vi "Do Start.vi"(6 "Diagnostics Queue":refnum<queue>, 7 "Host Resources":T1, 8 "error in":errorcluster, 10 "Generated Data":string, 11 "Hardware Configuration in":T5) -> (0 "error out":errorcluster, 2 "Acquired Data":T4, 3 "Hardware Configuration out":T5)   [LabVIEW 2021, in "Load Frame.lvlib"]
doc: "Configure DAQmx tasks to take measurements from the Load Frame sensors using the settings from 'Hardware Configuration in'."
uses:
  Load Frame.lvlib
  Acquisition/Hardware Configuration.ctl
  Acquisition/Channel Settings.ctl
  Acquisition/IO Device.ctl
  Acquisition/Sensor Type.ctl
  Interval Timer/Repeat Interval.ctl
  Interval Timer/Interval Length.ctl
  Interval Timer/Interval Token.ctl
  Acquisition/IO Context.ctl
  Acquisition/IO API.ctl
  Acquisition/Acquired Data.ctl
  Acquisition/Host Resources.ctl
  Acquisition/Host Software Package.ctl
  Acquisition/Host IO Resource.ctl
  support/Message Queue/Message Cluster.ctl
  74e49535-f2c9-4e2d-86ae-5e165b5420e6.vi
  c62da056-855e-47fb-b67a-8cab6a77d309.vi
  support/Message Queue/Enqueue Message (Single).vi
  support/Message Queue/Message Queue.lvlib
  Acquisition/Acquisition.lvlib
  Interval Timer/Interval Timer.lvlib
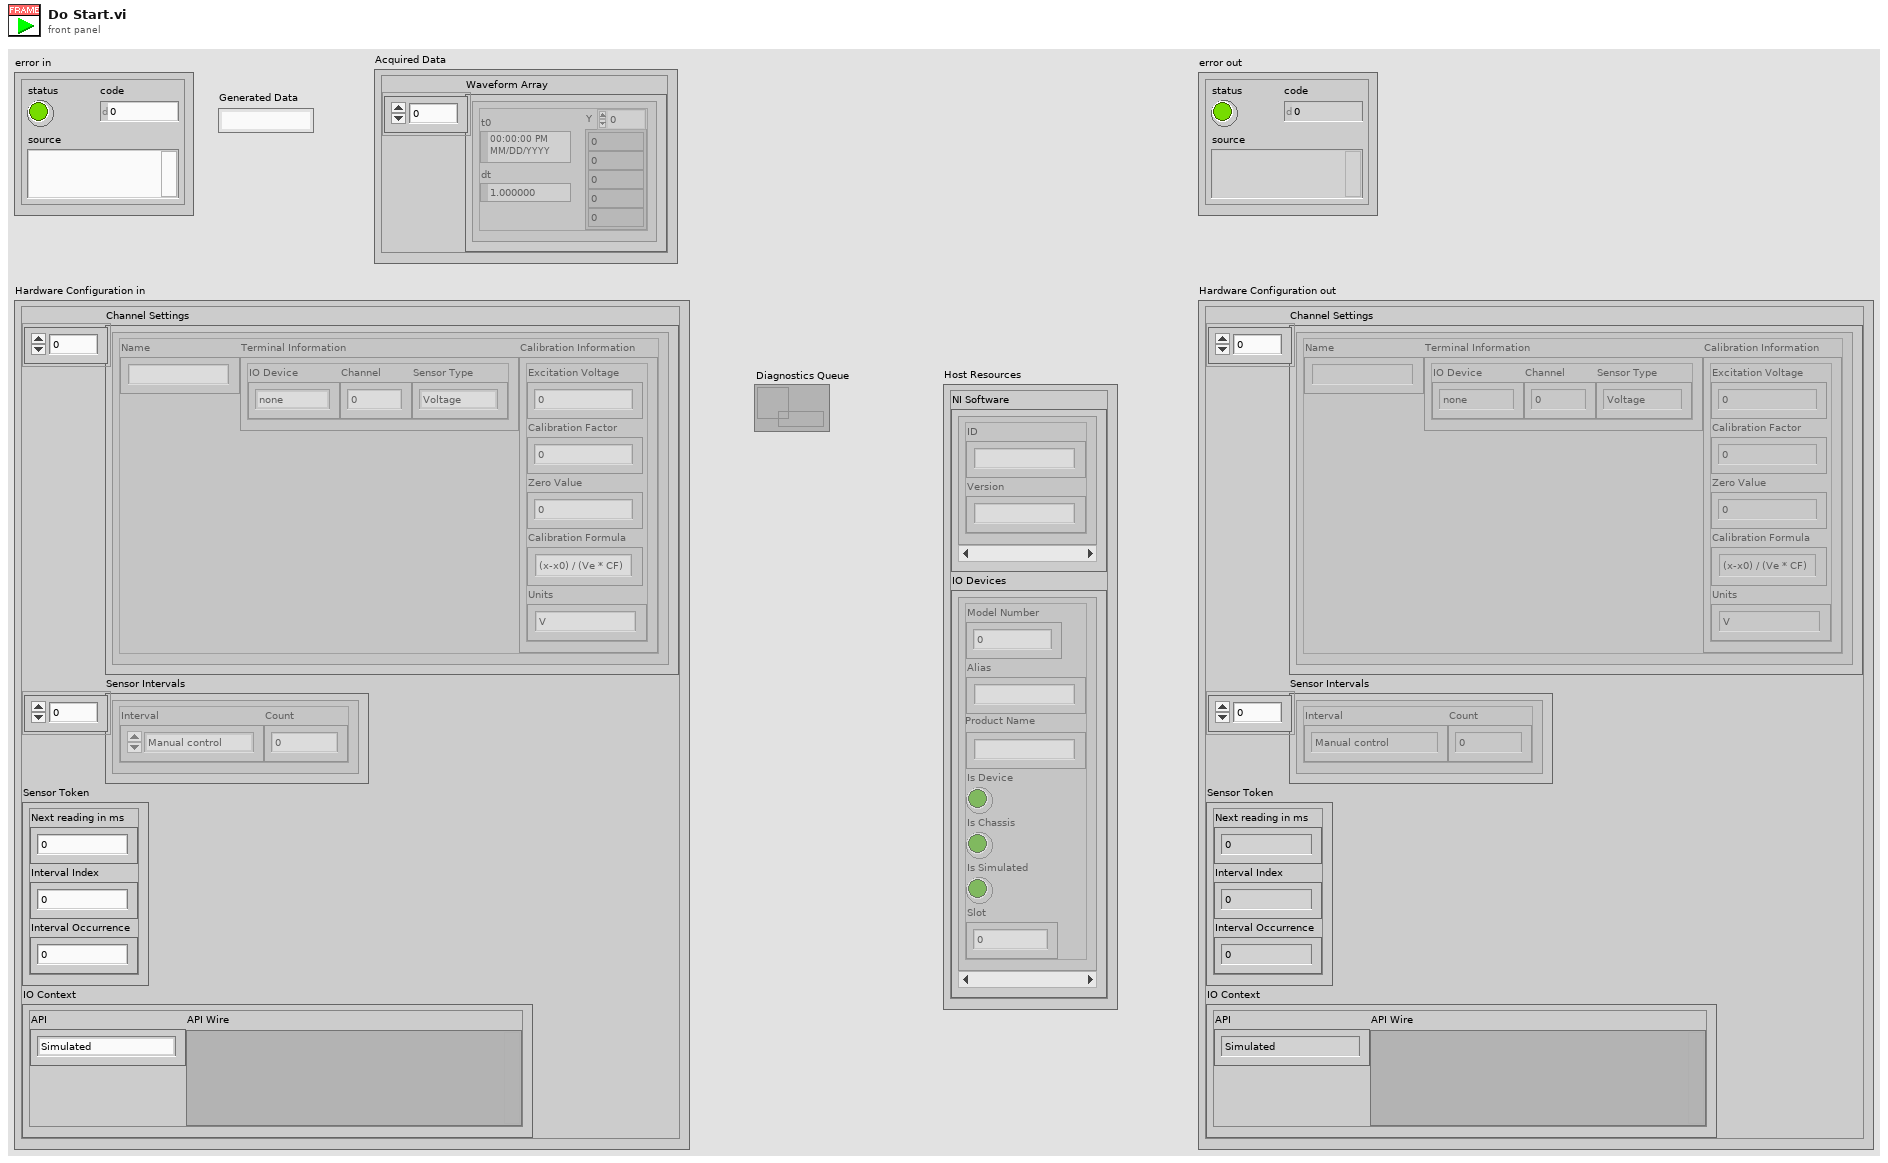
[diagram p1: front panel]
types:
  T1 = typedef "Acquisition.lvlib/Host Resources.ctl" = cluster{"NI Software":T2[], "IO Devices":T3[]}
  T2 = typedef "Acquisition.lvlib/Host Software Package.ctl" = cluster{"ID":string, "Version":string}
  T3 = typedef "Acquisition.lvlib/Host IO Resource.ctl" = cluster{"Model Number":u32, "Alias":string, "Product Name":string, "Is Device":bool, "Is Chassis":bool, "Is Simulated":bool, "Slot":i32}
  T4 = typedef "Acquisition.lvlib/Acquired Data.ctl" = cluster{"Waveform Array":waveform(dbl)[]}
  T5 = typedef "Acquisition.lvlib/Hardware Configuration.ctl" = cluster{"Channel Settings":T6[], "Sensor Intervals":T9[], "Sensor Token":T11, "IO Context":T12}
  T6 = typedef "Acquisition.lvlib/Channel Settings.ctl" = cluster{"Name":string, "Terminal Information":cluster{"IO Device":T7, "Channel":i32, "Sensor Type":T8}, "Calibration Information":cluster{"Excitation Voltage":dbl, "Calibration Factor":dbl, "Zero Value":dbl, "Calibration Formula":string, "Units":string}}
  T7 = typedef "Acquisition.lvlib/IO Device.ctl" = enum16{"none", "9219", "9401"}
  T8 = typedef "Acquisition.lvlib/Sensor Type.ctl" = enum16{"Voltage", "Load", "Pressure", "Encoder"}
  T9 = typedef "Interval Timer.lvlib/Repeat Interval.ctl" = cluster{"Interval":T10, "Count":i32}
  T10 = typedef "Interval Timer.lvlib/Interval Length.ctl" = enum16{"Manual control", "1 second", "10 seconds", "30 seconds", "60 seconds", "600 seconds", "1200 seconds", "3600 seconds"}
  T11 = typedef "Interval Timer.lvlib/Interval Token.ctl" = cluster{"Next reading in ms":u32, "Interval Index":i32, "Interval Occurrence":i32}
  T12 = typedef "Acquisition.lvlib/IO Context.ctl" = cluster{"API":T13, "API Wire":variant}
  T13 = typedef "Acquisition.lvlib/IO API.ctl" = enum16{"Simulated", "DAQmx"}
  T14 = cluster{"Timing Settings":string, "Channels":string[]}
  T15 = cluster{string, cluster{"Timing Settings":string, "Channels":string[]}[]}
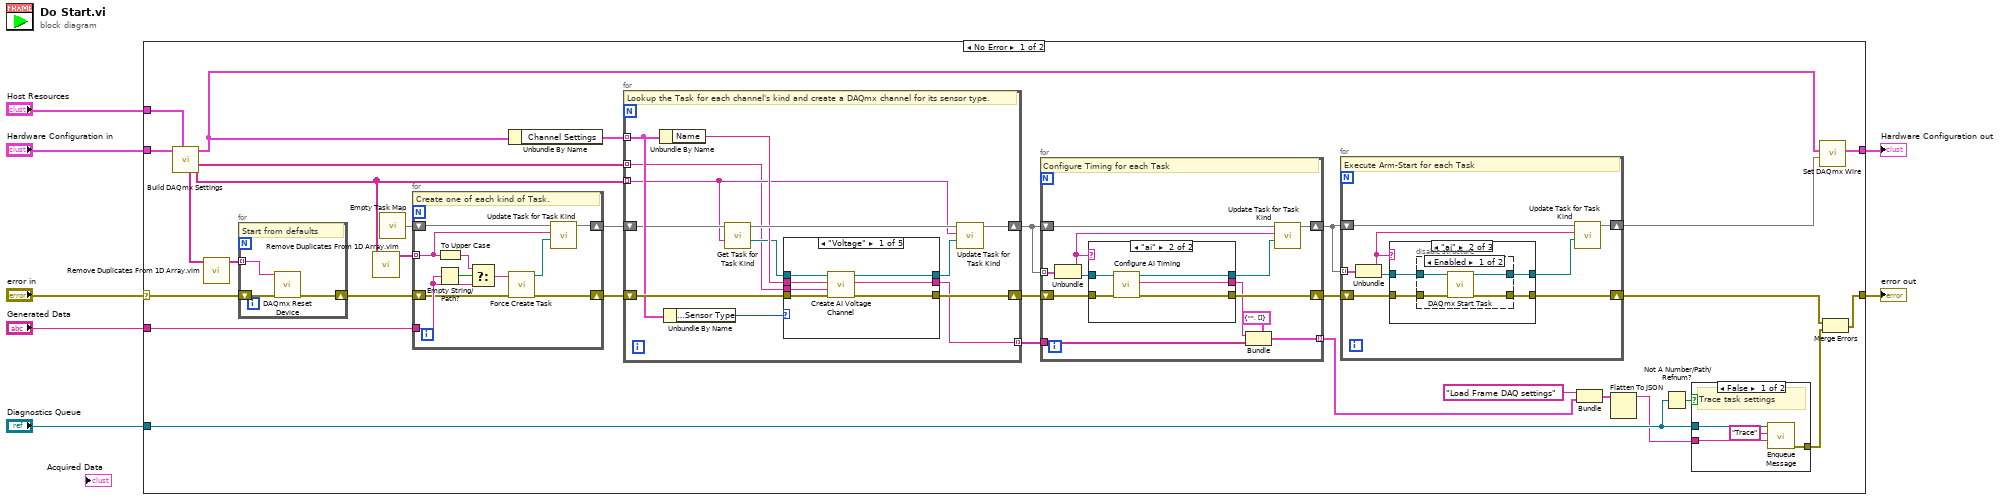
[diagram p0: block diagram]
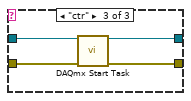
[diagram p4: hidden frame]
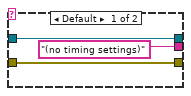
[diagram p5: hidden frame]
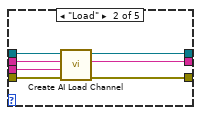
[diagram p6: hidden frame]
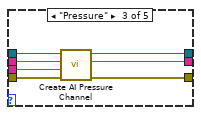
[diagram p7: hidden frame]
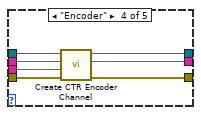
[diagram p8: hidden frame]
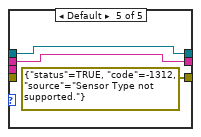
[diagram p9: hidden frame]
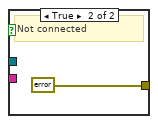
[diagram p10: hidden frame]
diagram:
  n1 = case shown="No Error" "error in" {
    selector: "error in" -> [w17 w146]
    tunnel: [w38 w145] -> w7
    tunnel: [w33 w146] -> w6
    tunnel: "Generated Data" -> [w15 _]
    tunnel: "Diagnostics Queue" -> [w34 _]
    tunnel: "Host Resources" -> [w29 _]
    tunnel: "Hardware Configuration in" -> [w28 w145]
    frame No Error {
      n2 = call "Build DAQmx Settings.vi"("Host Resources"=w29, "Hardware Configuration in"=w28) -> ("DAQ Task Kinds"=w26:string[], "Physical Channels"=w13:string[], "Hardware Configuration in out"=w27:T5, "DAQ Device Names"=w12:string[])  [unwired: 6 in]
      n3 = call "Remove Duplicates From 1D Array.vim"("array"=w12) -> ("array with duplicates removed"=w18:string[])  [unwired: 10 in]
      n4 = for {
        tunnel: w18 -> [w41] mode=indexing
        shift-right: [w39] -> w16
        shift-left: w17 -> [w40]
        # "Start from defaults"
        n5 = call <vilib>:"DAQmx Reset Device.vi"("device in"=w41, "error in"=w40) -> ("error out"=w39:errorcluster)  [unwired: 13 in]
      }
      n6 = call "Remove Duplicates From 1D Array.vim"("array"=w26) -> ("array with duplicates removed"=w31:string[])  [unwired: 10 in]
      n7 = call "Empty Task Map.vi"() -> ("Task Map"=w25:map{string, refnum<k21>})
      n8 = for {
        tunnel: w15 -> [w138]
        shift-right: [w135] -> w14
        shift-left: w16 -> [w137]
        tunnel: w31 -> [w130] mode=indexing
        shift-right: [w133] -> w24
        shift-left: w25 -> [w134]
        # "Create one of each kind of Task."
        n9 = Empty String/Path?(string/path=w138) -> (empty?=w139:bool)
        n10 = To Upper Case(1:w130) -> (0:w136:string)
        n11 = Select(t=w136, s=w139, f=w138) -> (s? t:f=w132:string)
        n12 = call "Force Create Task.vi"("error in (no error)"=w137, "Task Name"=w132) -> ("error out"=w135:errorcluster, "Task out"=w131:refnum<k21>)  [unwired: 8 in]
        n13 = call "Update Task for Task Kind.vi"("DAQmx Task"=w131, "DAQmx Task prefix"=w130, "Task Map in"=w134) -> ("Task Map out"=w133:map{string, refnum<k21>})  [unwired: 8 in]
      }
      n14 = Unbundle By Name(w27) -> ("Channel Settings"=w36:T6[])
      n15 = for {
        tunnel: w36 -> [w94] mode=indexing
        shift-right: [w98] -> w37
        shift-left: w14 -> [w95]
        tunnel: w26 -> [w87] mode=indexing
        tunnel: [w96] -> w30 mode=indexing
        shift-right: [w88] -> w23
        shift-left: w24 -> [w90]
        tunnel: w13 -> [w86] mode=indexing
        # "Lookup the Task for each channel's kind and create a DAQmx channel for its sensor type."
        n16 = Unbundle By Name(w94) -> ("Name"=w92:string)
        n17 = Unbundle By Name(w94) -> ("Terminal Information.Sensor Type"=w93:T8)
        n18 = call "Get Task for Task Kind.vi"("DAQmx Task prefix"=w87, "Task Map in"=w90) -> ("DAQmx Task"=w89:refnum<k21>, "Task Map out"=w97:map{string, refnum<k21>})  [unwired: 7 in, 1 out]
        n19 = case shown="\"Voltage\"" w93 {
          tunnel: w89 -> [w105 w112 w119 w124 w129]
          tunnel: [w103 w110 w117 w123 w129] -> w91
          tunnel: [w104 w111 w118 w125 errorcluster {"status"=TRUE, "code"=-1312, "source"="Sensor Type not supported."} ("error IO")] -> w98
          tunnel: w86 -> [w101 w108 w115 w120 _]
          tunnel: w95 -> [w102 w109 w116 w126 _]
          tunnel: [w100 w107 w114 w121 w128] -> w96
          tunnel: w92 -> [w99 w106 w113 w122 w128]
          frame "Voltage" {
            n20 = call "Create AI Voltage Channel.vi"("error in (no error)"=w102, "Physical channel"=w101, "Name"=w99, "Task in"=w105) -> ("error out"=w104:errorcluster, "Voltage Channel Settings"=w100:string, "Task out"=w103:refnum<k21>)  [unwired: 5 in]
          }
          frame "Load" {
            n21 = call "Create AI Load Channel.vi"("error in (no error)"=w109, "Physical Channel"=w108, "Name"=w106, "Task in"=w112) -> ("error out"=w111:errorcluster, "Load Channel Settings"=w107:string, "Task out"=w110:refnum<k21>)  [unwired: 5 in]
          }
          frame "Pressure" {
            n22 = call "Create AI Pressure Channel.vi"("error in (no error)"=w116, "Physical channel"=w115, "Name"=w113, "Task in"=w119) -> ("error out"=w118:errorcluster, "Pressure Channel Settings"=w114:string, "Task out"=w117:refnum<k21>)  [unwired: 5 in]
          }
          frame "Encoder" {
            n23 = call "Create CTR Encoder Channel.vi"("error in (no error)"=w126, "Physical channel"=w120, "Name"=w122, "Task in"=w124) -> ("error out"=w125:errorcluster, "Encoder Channel Settings"=w121:string, "Task out"=w123:refnum<k21>)  [unwired: 5 in]
          }
          frame Default {
          }
        }
        n24 = call "Update Task for Task Kind.vi"("DAQmx Task"=w91, "DAQmx Task prefix"=w87, "Task Map in"=w97) -> ("Task Map out"=w88:map{string, refnum<k21>})  [unwired: 8 in]
      }
      n25 = for {
        tunnel: [w75] -> w8 mode=indexing
        tunnel: w30 -> [w74]
        shift-right: [w76] -> w21
        shift-left: w37 -> [w77]
        tunnel: w23 -> [w72] mode=indexing
        shift-right: [w68] -> w19
        shift-left: w23 -> [w69]
        # "Configure Timing for each Task"
        n26 = Unbundle(w72) -> (w66:string, w71:refnum<k21>)
        n27 = case shown="\"ai\"" w66 {
          tunnel: w77 -> [w79 w85]
          tunnel: [w79 w84] -> w76
          tunnel: [w80 w83] -> w67
          tunnel: ["(no timing settings)" ("AI Timing Settings") w82] -> w73
          tunnel: w71 -> [w80 w81]
          frame Default {
          }
          frame "ai" {
            n28 = call "Configure AI Timing.vi"("error in (no error)"=w85, "Task in"=w81) -> ("error out"=w84:errorcluster, "AI Timing Settings"=w82:string, "Task out"=w83:refnum<k21>)  [unwired: 7 in]
          }
        }
        n29 = Bundle(cluster=T14 {"Timing Settings"="", "Channels"=[]} ("Task Settings"), "Timing Settings"=w73, "Channels"=w74) -> (w75:T14)
        n30 = call "Update Task for Task Kind.vi"("DAQmx Task"=w67, "DAQmx Task prefix"=w66, "Task Map in"=w69) -> ("Task Map out"=w68:map{string, refnum<k21>})  [unwired: 8 in]
      }
      n31 = for {
        shift-right: [w42] -> w20
        shift-left: w21 -> [w49]
        tunnel: w19 -> [w48] mode=indexing
        shift-right: [w45] -> w22
        shift-left: w19 -> [w46]
        # "Execute Arm-Start for each Task"
        n32 = Unbundle(w48) -> (w43:string, w47:refnum<k21>)
        n33 = case shown="\"ai\"" w43 {
          tunnel: w49 -> [w50 w54 w65]
          tunnel: [w50 w52 w64] -> w42
          tunnel: [w51 w53 w62] -> w44
          tunnel: w47 -> [w51 w55 w63]
          frame Default {
          }
          frame "ai" {
            n34 = disable-structure shown="Enabled" {
              disable-tunnel: w55 -> [w59 w61]
              disable-tunnel: w54 -> [w58 w60]
              disable-tunnel: [w57 w61] -> w53
              disable-tunnel: [w56 w60] -> w52
              frame Enabled {
                n35 = call <vilib>:"DAQmx Start Task.vi"("task/channels in"=w59, "error in"=w58) -> ("task out"=w57:refnum<k21>, "error out"=w56:errorcluster)  [unwired: 12 in]
              }
              frame Disabled {
              }
            }
          }
          frame "ctr" {
            n36 = call <vilib>:"DAQmx Start Task.vi"("task/channels in"=w63, "error in"=w65) -> ("task out"=w62:refnum<k21>, "error out"=w64:errorcluster)  [unwired: 12 in]
          }
        }
        n37 = call "Update Task for Task Kind.vi"("DAQmx Task"=w44, "DAQmx Task prefix"=w43, "Task Map in"=w46) -> ("Task Map out"=w45:map{string, refnum<k21>})  [unwired: 8 in]
      }
      n38 = Bundle("Load Frame DAQ settings", w8) -> (w10:T15)  [unwired: 1 in]
      n39 = Flatten To JSON(anything=w10) -> (JSON string=w11:string)  [unwired: 2 in, 1 out]
      n40 = Not A Number/Path/Refnum?(number/path/refnum=w34) -> (NaN/Path/Refnum?=w35:bool)
      n41 = case shown="False" w35 {
        tunnel: w34 -> [w143 _]
        tunnel: [w141 errorcluster {"status"=FALSE, "code"=0, "source"=""} ("error out")] -> w32
        tunnel: w11 -> [w140 _]
        frame False {
          # "Trace task settings"
          n42 = call-poly "Enqueue Message.vi"("Message Data"=w140, "Message"="Trace", "Message Queue"=w143) -> ("error out"=w141:errorcluster)  [unwired: 7 in, 1 out]
        }
        frame True {
          # "Not connected"
        }
      }
      n43 = call "Set DAQmx Wire.vi"("Task Map"=w22, "Hardware Configuration"=w27) -> ("Hardware Configuration out"=w38:T5)  [unwired: 7 in]
      n44 = Merge Errors(w20, w32) -> (w33:errorcluster)
    }
    frame Error {
    }
  }
  "Hardware Configuration out" <- w7
  "error out" <- w6
